vi "handle_CAN_error.vi"(11 "error in (no error)":errorcluster) -> (1 "stop":bool, 3 "error out":errorcluster)   [LabVIEW 2020]
uses:
  <vilib>/ErrorRing/Error Ring.xnode
panel:
  in  "retry delay (ms)":u32=300
  in  "# of tries":i32=3
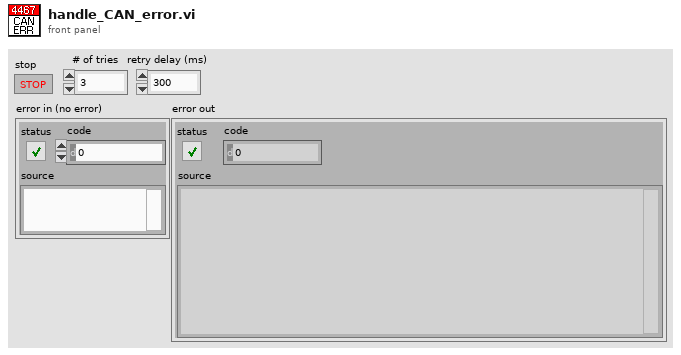
[diagram p1: front panel]
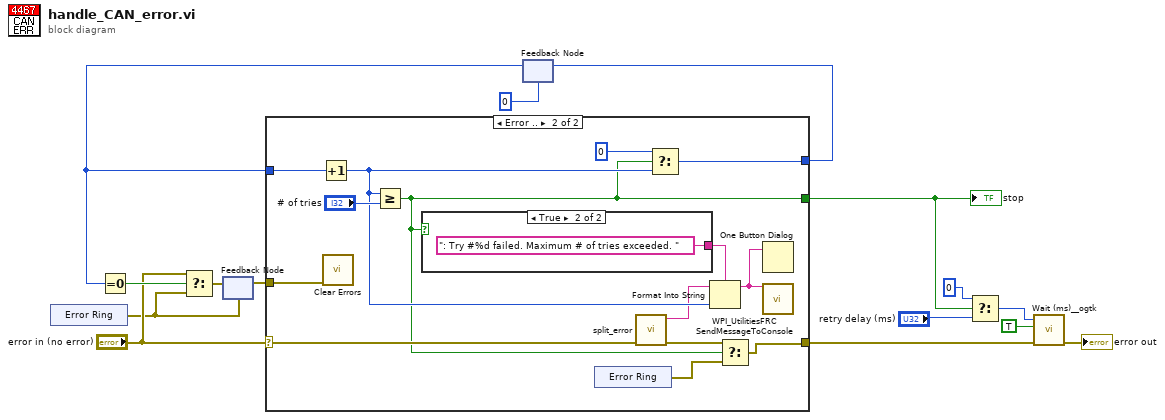
[diagram p0: block diagram]
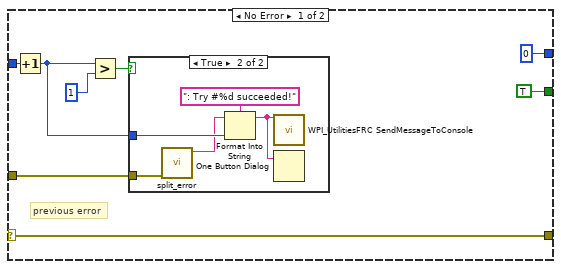
[diagram p2: hidden frame]
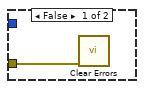
[diagram p3: hidden frame]
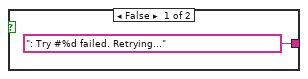
[diagram p4: hidden frame]
diagram:
  n1 = xnode "Error Ring"() -> ("error out"=w3:errorcluster)
  n2 = feedback #1(w3) -> (w1:errorcluster)
  n3 = feedback #2(0) -> (w6:i32)
  n4 = Equal To 0?(x=w6) -> (x = 0?=w5:bool)
  n5 = Select(t="error in (no error)", s=w5, f=w3) -> (s? t:f=w2:errorcluster)
  n6 = feedback-in #1(w2) -> ()
  n7 = case shown="Error .." "error in (no error)" {
    selector: "error in (no error)" -> [w21 w36]
    tunnel: w6 -> [w20 w43]
    tunnel: [0 w40] -> w14
    tunnel: [TRUE ("stop") w33] -> w12
    tunnel: [w21 w30] -> w10
    tunnel: w1 -> [w17 w39]
    frame No Error {
      # "previous error"
      n8 = Increment(x=w20) -> (x+1=w18:i32)
      n9 = Greater?(x=w18, y=1) -> (0:w16:bool)
      n10 = case shown="True" w16 {
        tunnel: w18 -> [_ w29]
        tunnel: w17 -> [w24 w27]
        frame False {
          n11 = call <vilib>:"Clear Errors.vi"("error in (no error)"=w24) -> ()  [unwired: 5 in, 2 out]
        }
        frame True {
          n12 = call "split_error.vi"("error in"=w27) -> ("Details"=w26:string)  [unwired: 7 in, 3 out]
          n13 = Format Into String(format string=": Try #%d succeeded!" ("message"), initial string=w26, w29) -> (resulting string=w25:string)  [unwired: 1 in, 1 out]
          n14 = call <vilib>:"WPI_UtilitiesFRC SendMessageToConsole.vi"("Message"=w25) -> ()  [unwired: 14 in, 1 out]
          n15 = One Button Dialog(message=w25) -> ()  [unwired: 1 in, 1 out]
        }
      }
    }
    frame Error {
      n16 = Increment(x=w43) -> (x+1=w38:i32)
      n17 = call <vilib>:"Clear Errors.vi"("error in (no error)"=w39) -> ()  [unwired: 5 in, 2 out]
      n18 = Greater Or Equal?(x=w38, y="# of tries") -> (x >= y?=w33:bool)
      n19 = case shown="True" w33 {
        tunnel: [": Try #%d failed. Retrying..." ("message") ": Try #%d failed. Maximum # of tries exceeded. " ("message")] -> w37
        frame False {
        }
        frame True {
        }
      }
      n20 = xnode "Error Ring"() -> ("error out"=w31:errorcluster)
      n21 = call "split_error.vi"("error in"=w36) -> ("error out"=w32:errorcluster, "Details"=w35:string)  [unwired: 7 in, 2 out]
      n22 = Select(t=0, s=w33, f=w38) -> (s? t:f=w40:i32)
      n23 = Format Into String(format string=w37, initial string=w35, w38) -> (resulting string=w34:string)  [unwired: 1 in, 1 out]
      n24 = Select(t=w32, s=w33, f=w31) -> (s? t:f=w30:errorcluster)
      n25 = One Button Dialog(message=w34) -> ()  [unwired: 1 in, 1 out]
      n26 = call <vilib>:"WPI_UtilitiesFRC SendMessageToConsole.vi"("Message"=w34) -> ()  [unwired: 14 in, 1 out]
    }
  }
  "stop" <- w12
  n27 = feedback-in #2(w14) -> ()
  n28 = Select(t=u32 0, s=w12, f="retry delay (ms)") -> (s? t:f=w7:u32)
  n29 = call "Wait (ms)__ogtk.vi"("error in (no error)"=w10, "Wait on Error (FALSE)"=TRUE, "milliseconds to wait"=w7) -> ("error out"=→"error out":errorcluster)  [unwired: 7 in, 1 out]
